vi "Determine Value Source.vi"(8 "error in (no error)":errorcluster, 11 "Composed Column Factory in":refnum<class "Composed Column Factory.lvclass">) -> (0 "error out":errorcluster, 2 "Value Source":refnum<class "Value Source.lvclass">, 3 "Composed Column Factory out":refnum<class "Composed Column Factory.lvclass">)   [LabVIEW 2020, in "Composed Columns.lvlib" / "Composed Column Factory.lvclass"]
uses:
  Composed Column Factory.lvclass
  Composed Columns/Value Source Interface Class/Value Source.lvclass
  Value Source/Variant Value Source.lvclass
  C:/Users/User/Desktop/Raman Program/Database OOP/source/Database OOP/Column Libraries/Composed Columns/Value Source Interface Class/Value Source.lvclass
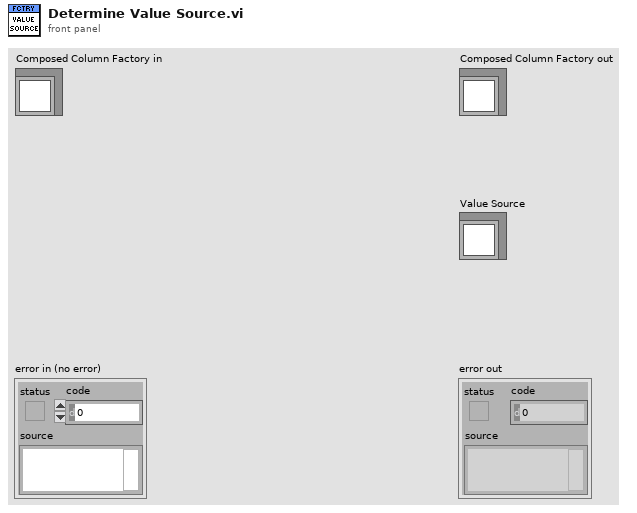
[diagram p1: front panel]
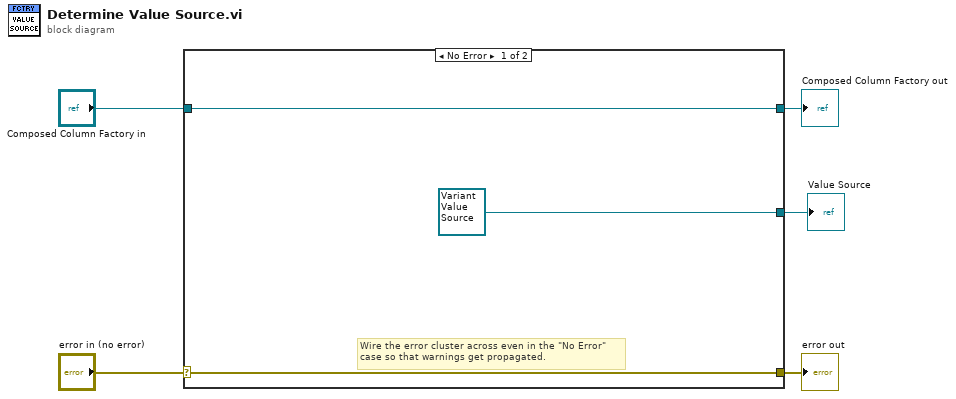
[diagram p0: block diagram]
diagram:
  n1 = case shown="No Error" "error in (no error)" {
    selector: "error in (no error)" -> [w7 w10]
    tunnel: [w7 w10] -> w4
    tunnel: [w8 w9] -> w2
    tunnel: "Composed Column Factory in" -> [w8 w9]
    tunnel: [refnum<class "Variant Value Source.lvclass"> refnum ("Composed Columns.lvlib:Variant Value Source.lvclass") _] -> w1
    frame No Error {
      # "Wire the error cluster across even in the \"No Error\"\ncase so that warnings get propagated."
    }
    frame Error {
    }
  }
  "error out" <- w4
  "Composed Column Factory out" <- w2
  "Value Source" <- w1
